vi "test_write.vi"() -> ()   [LabVIEW 2014]
uses:
  nii_read_head.vi
  nii_write.vi
panel:
  in  "save":bool
  in  "datatype":string
  in  "index (page)":i32=20
  in  "stop":bool
  out "new picture":picture
  in  "nii_write":path
  in  "nii_source":path
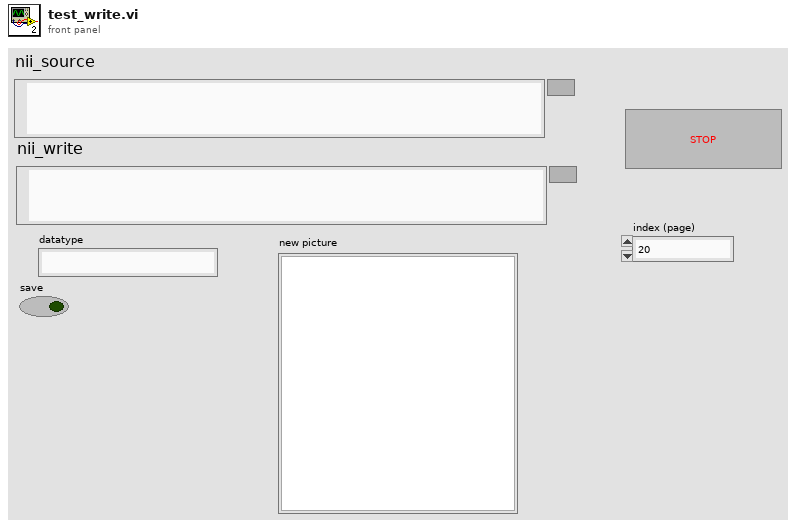
[diagram p1: front panel]
types:
  T1 = typedef "head_data.ctl" = cluster{"hdr size":i32, "dim":i32[], "data bit size":i32, "datatype":string, "pixel size ":sgl[], "voxel offset":sgl, "range of calibration values-max,min":sgl[], " pixel values- max, min":sgl[], "slice orientation":u16}
  T2 = typedef "imagedata.ctl" = cluster{"image type":i32, "image depth":i32, "image":u8[], "mask":u8[], "colors":u32[], "Rectangle":cluster{"left":i16, "top":i16, "right":i16, "bottom":i16}}
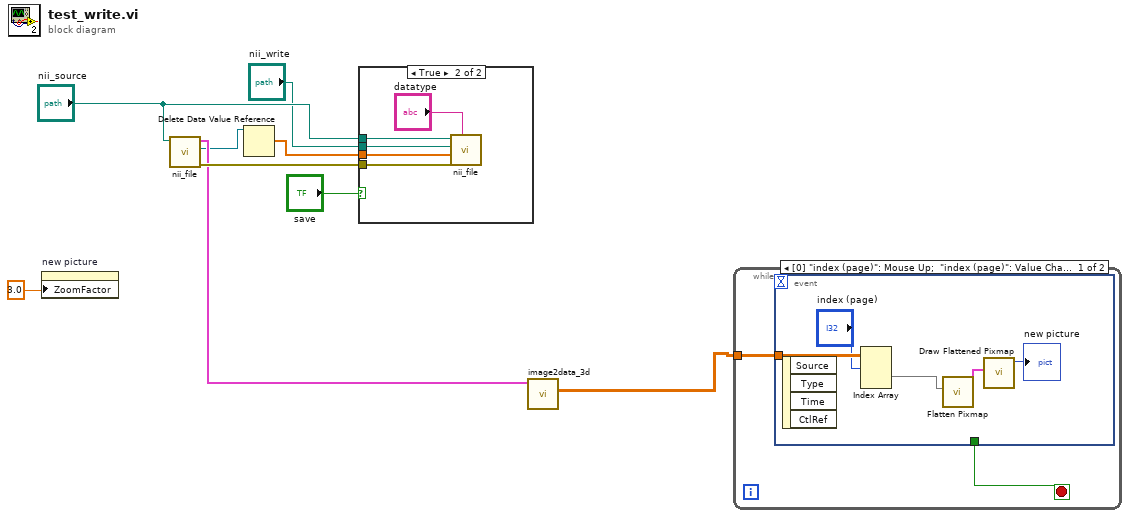
[diagram p0: block diagram]
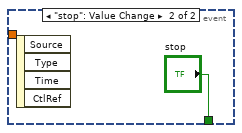
[diagram p3: hidden frame]
diagram:
  n1 = property on="new picture" class="Pict"("ZoomFactor"=sgl 3.0 ("Zoom Factor")) -> ()  [unwired: 2 in, 2 out]
  n2 = call-poly "nii_file.vi"("file (use dialog)"="nii_source") -> ("error out"=w8:errorcluster, "data value reference"=w2:refnum<data-value>, "Data"=w6:T1)  [unwired: 6 in, 2 out]
  n3 = Delete Data Value Reference(data value reference=w2) -> (data value=w1:cdb[])  [unwired: 1 in, 1 out]
  n4 = case shown="True" "save" {
    tunnel: "nii_source" -> [_ w14]
    tunnel: w8 -> [_ w13]
    tunnel: "nii_write" -> [_ w12]
    tunnel: w1 -> [_ w10]
    frame False {
    }
    frame True {
      n5 = call-poly "nii_file.vi"("datatype"="datatype", "error in (no error)"=w13, "data in"=w10, "nii_write"=w12, "nii_source"=w14) -> ()  [unwired: 6 in, 1 out]
    }
  }
  n6 = call "image2data_3d.vi"("Data"=w6) -> ("imag3_3d"=w3:sgl[][][])  [unwired: 9 in, 1 out]
  n7 = while {
    tunnel: w3 -> [w16]
    stop <- w15 stop-if-true
    n8 = event shown="[0] \"index (page)\": Mouse Up;  \"index (page)\": Value Change" {
      selector: _ -> [_ _]
      dyn-events: _ -> [_ _]
      timeout: _ -> [_ _]
      tunnel: w16 -> [w21 _]
      tunnel: [_ "stop"] -> w15
      event "index (page)": Mouse Up; "index (page)": Value Change {
        n9 = event-data() -> ()  [unwired: 1 in, 4 out]
        n10 = Index Array(array=w21, index (dim 0)="index (page)") -> (element=w17:sgl[][])  [unwired: 2 in]
        n11 = call <vilib>:"Flatten Pixmap.vi"("8-bit pixmap"=w17) -> ("image data"=w19:T2)  [unwired: 10 in]
        n12 = call <vilib>:"Draw Flattened Pixmap.vi"("image data"=w19) -> ("new picture"=→"new picture":picture)  [unwired: 8 in]
      }
      event "stop": Value Change {
        n13 = event-data() -> ()  [unwired: 1 in, 4 out]
      }
    }
  }
